vi "7L17-penalite_init_0.vi"(1 "Ccpc":dbl, 2 "Cc":dbl) -> (0 "Ccpc init":dbl)   [LabVIEW 2010, in "lv_07.lvlib"]
doc: "Si le Coût d'une commande en urgence (Ccpc) est <=0 alors, il est initialisé à la valeur d'une commande normale (Cc)"
uses:
  lv_07.lvlib
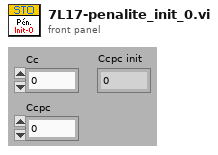
[diagram p1: front panel]
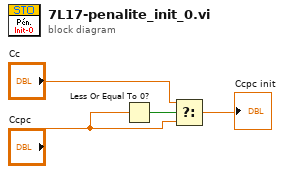
[diagram p0: block diagram]
diagram:
  n1 = Less Or Equal To 0?(x="Ccpc") -> (x <= 0?=w3:bool)
  n2 = Select(t="Cc", s=w3, f="Ccpc") -> (s? t:f=→"Ccpc init":dbl)
